vi "Connect.vi"(8 "error in (no error)":errorcluster, 10 "Data Source":string, 11 "PostgreSQL in":refnum<class "PostgreSQL.lvclass">) -> (0 "error out":errorcluster, 3 "PostgreSQL out":refnum<class "PostgreSQL.lvclass">)   [LabVIEW 2018, in "Database.lvlib" / "PostgreSQL.lvclass"]
uses:
  PostgreSQL.lvclass
  DatabaseBaseClass/DatabaseBaseClass.lvclass
panel:
  # "Connecting to Database..."
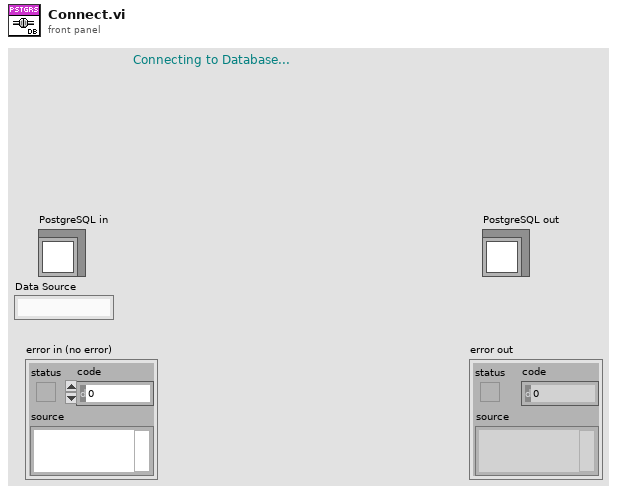
[diagram p1: front panel]
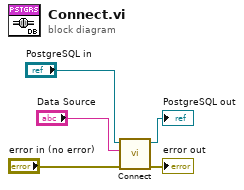
[diagram p0: block diagram]
diagram:
  n1 = call-parent "Connect.vi"("error in (no error)"="error in (no error)", "Data Source"="Data Source", "DatabaseBaseClass in"="PostgreSQL in") -> ("error out"=→"error out":errorcluster, "DatabaseBaseClass out"=→"PostgreSQL out":refnum<class "PostgreSQL.lvclass">)  [unwired: 7 in]
